vi "pressure delta.vi"(11 "unsigned byte array":u8[](array[numeric])) -> (0 "x-y 4":dbl, 1 "x-y 3":dbl, 2 "x-y 2":dbl, 3 "x-y 1":dbl, 5 "x-y  5":dbl)   [LabVIEW 2016]
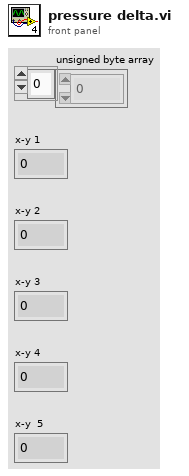
[diagram p1: front panel]
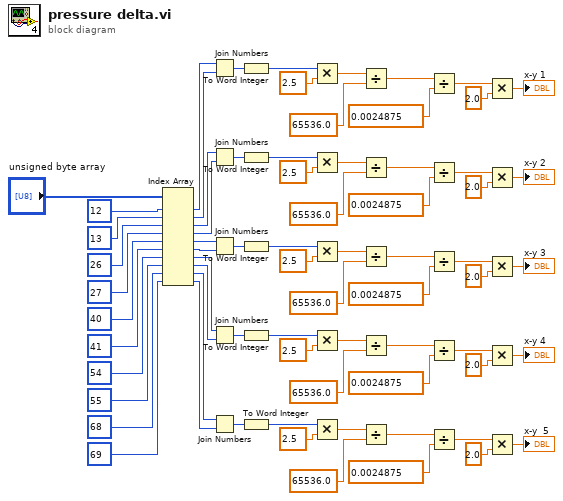
[diagram p0: block diagram]
diagram:
  n1 = Index Array(array="unsigned byte array", index #1=12 ("index"), index #2=13 ("index"), index #3=26 ("index"), index #4=27 ("index"), index #5=40 ("index"), index #6=41 ("index"), index #7=54 ("index"), index #8=55 ("index"), index #9=68 ("index"), index #10=69 ("index")) -> (element #1=w18:u8, element #2=w19:u8, element #3=w49:u8, element #4=w48:u8, element #5=w42:u8, element #6=w41:u8, element #7=w35:u8, element #8=w34:u8, element #9=w56:u8, element #10=w55:u8)
  n2 = Join Numbers(hi=w18, lo=w19) -> ((hi.lo)=w17:u16)
  n3 = Join Numbers(hi=w49, lo=w48) -> ((hi.lo)=w27:u16)
  n4 = Join Numbers(hi=w42, lo=w41) -> ((hi.lo)=w24:u16)
  n5 = Join Numbers(hi=w35, lo=w34) -> ((hi.lo)=w22:u16)
  n6 = Join Numbers(hi=w56, lo=w55) -> ((hi.lo)=w20:u16)
  n7 = To Word Integer(number=w17) -> (16bit integer=w16:i16)
  n8 = To Word Integer(number=w27) -> (16bit integer=w26:i16)
  n9 = To Word Integer(number=w24) -> (16bit integer=w25:i16)
  n10 = To Word Integer(number=w22) -> (16bit integer=w23:i16)
  n11 = To Word Integer(number=w20) -> (16bit integer=w21:i16)
  n12 = Multiply(x=w16, y=2.5) -> (x*y=w33:dbl)
  n13 = Multiply(x=w26, y=2.5) -> (x*y=w54:dbl)
  n14 = Multiply(x=w25, y=2.5) -> (x*y=w47:dbl)
  n15 = Multiply(x=w23, y=2.5) -> (x*y=w40:dbl)
  n16 = Multiply(x=w21, y=2.5) -> (x*y=w61:dbl)
  n17 = Divide(x=w33, y=65536.0) -> (x/y=w31:dbl)
  n18 = Divide(x=w54, y=65536.0) -> (x/y=w52:dbl)
  n19 = Divide(x=w47, y=65536.0) -> (x/y=w45:dbl)
  n20 = Divide(x=w40, y=65536.0) -> (x/y=w38:dbl)
  n21 = Divide(x=w61, y=65536.0) -> (x/y=w59:dbl)
  n22 = Divide(x=w31, y=0.0024875) -> (x/y=w14:dbl)
  n23 = Divide(x=w52, y=0.0024875) -> (x/y=w11:dbl)
  n24 = Divide(x=w45, y=0.0024875) -> (x/y=w8:dbl)
  n25 = Divide(x=w38, y=0.0024875) -> (x/y=w5:dbl)
  n26 = Divide(x=w59, y=0.0024875) -> (x/y=w2:dbl)
  n27 = Multiply(x=w14, y=2.0) -> (x*y=→"x-y 1":dbl)
  n28 = Multiply(x=w11, y=2.0) -> (x*y=→"x-y 2":dbl)
  n29 = Multiply(x=w8, y=2.0) -> (x*y=→"x-y 3":dbl)
  n30 = Multiply(x=w5, y=2.0) -> (x*y=→"x-y 4":dbl)
  n31 = Multiply(x=w2, y=2.0) -> (x*y=→"x-y  5":dbl)
